vi "Channel Calibration.vi"(8 "error in (no error)":errorcluster, 9 "Gain":dbl, 10 "Channel Name":string, 11 "index":i32) -> (0 "error out":errorcluster, 1 "Offset":dbl, 2 "Gain":dbl, 3 "Status Output":T1)   [LabVIEW 2011]
uses:
  Calibration SubVIs/Controls/typedef_enum_Calibration Type.ctl
  Controls/typedef_enum_Calibration SM States.ctl
  Calibration SubVIs/Controls/typedef_enum_GFV Calibration GUI_actions.ctl
  Controls/typedef_cluster_Calibration Status.ctl
  Measurments Handling/Action Analog Handler.ctl
panel:
  out "Waveform Chart":dbl(graph)
  in  "Cancel":bool
  in  "OK":bool
  out "Instructions":string
  in  "Back":bool
  in  "Next":bool
  in  "Calibration Type":T2
  out "X2":dbl
  in  "Y2":dbl
  out "X1":dbl
  in  "Y1":dbl
  # "Channel Calibration"
  # "1st point"
  # "2nd point"
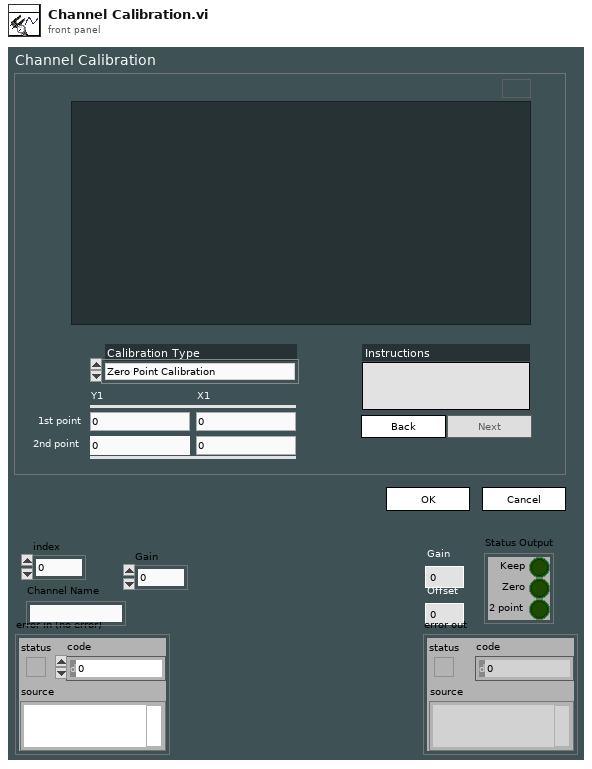
[diagram p1: front panel]
types:
  T1 = cluster{"Keep":bool, "Zero":bool, "2 point":bool}
  T2 = typedef "typedef_enum_Calibration Type.ctl" = enum16{"Zero Point Calibration", "Two Point Calibration"}
  T3 = typedef "typedef_cluster_Calibration Status.ctl" = cluster{"Keep":bool, "Zero":bool, "2 point":bool}
  T4 = typedef "typedef_enum_Calibration SM States.ctl" = enum16{"Idle", "Init", "2 pnt Enter 1st", "2 pnt Measure 1st", "2 pnt Enter 2nd", "2 pnt Measure 2nd", "2 pnt Calculate", "Zero Measure", "Zero Calculate", "Increment", "Decrement"}
  T5 = typedef "typedef_enum_GFV Calibration GUI_actions.ctl" = enum16{"Init", "Update GUI", "Clear GUI"}
  T6 = enum8{"Enabled", "Disabled", "Disabled and Grayed Out"}
  T7 = typedef "Action Analog Handler.ctl" = enum16{"GET value", "GET Single Frequenzy", "GET All Values", "GET Waveform", "Get Numb Var", "SET Value", "START Buffer", "REG Variable", "BUF size(total antal sekund)", "PULS", "Get a Value at time", "Set initial waveform"}
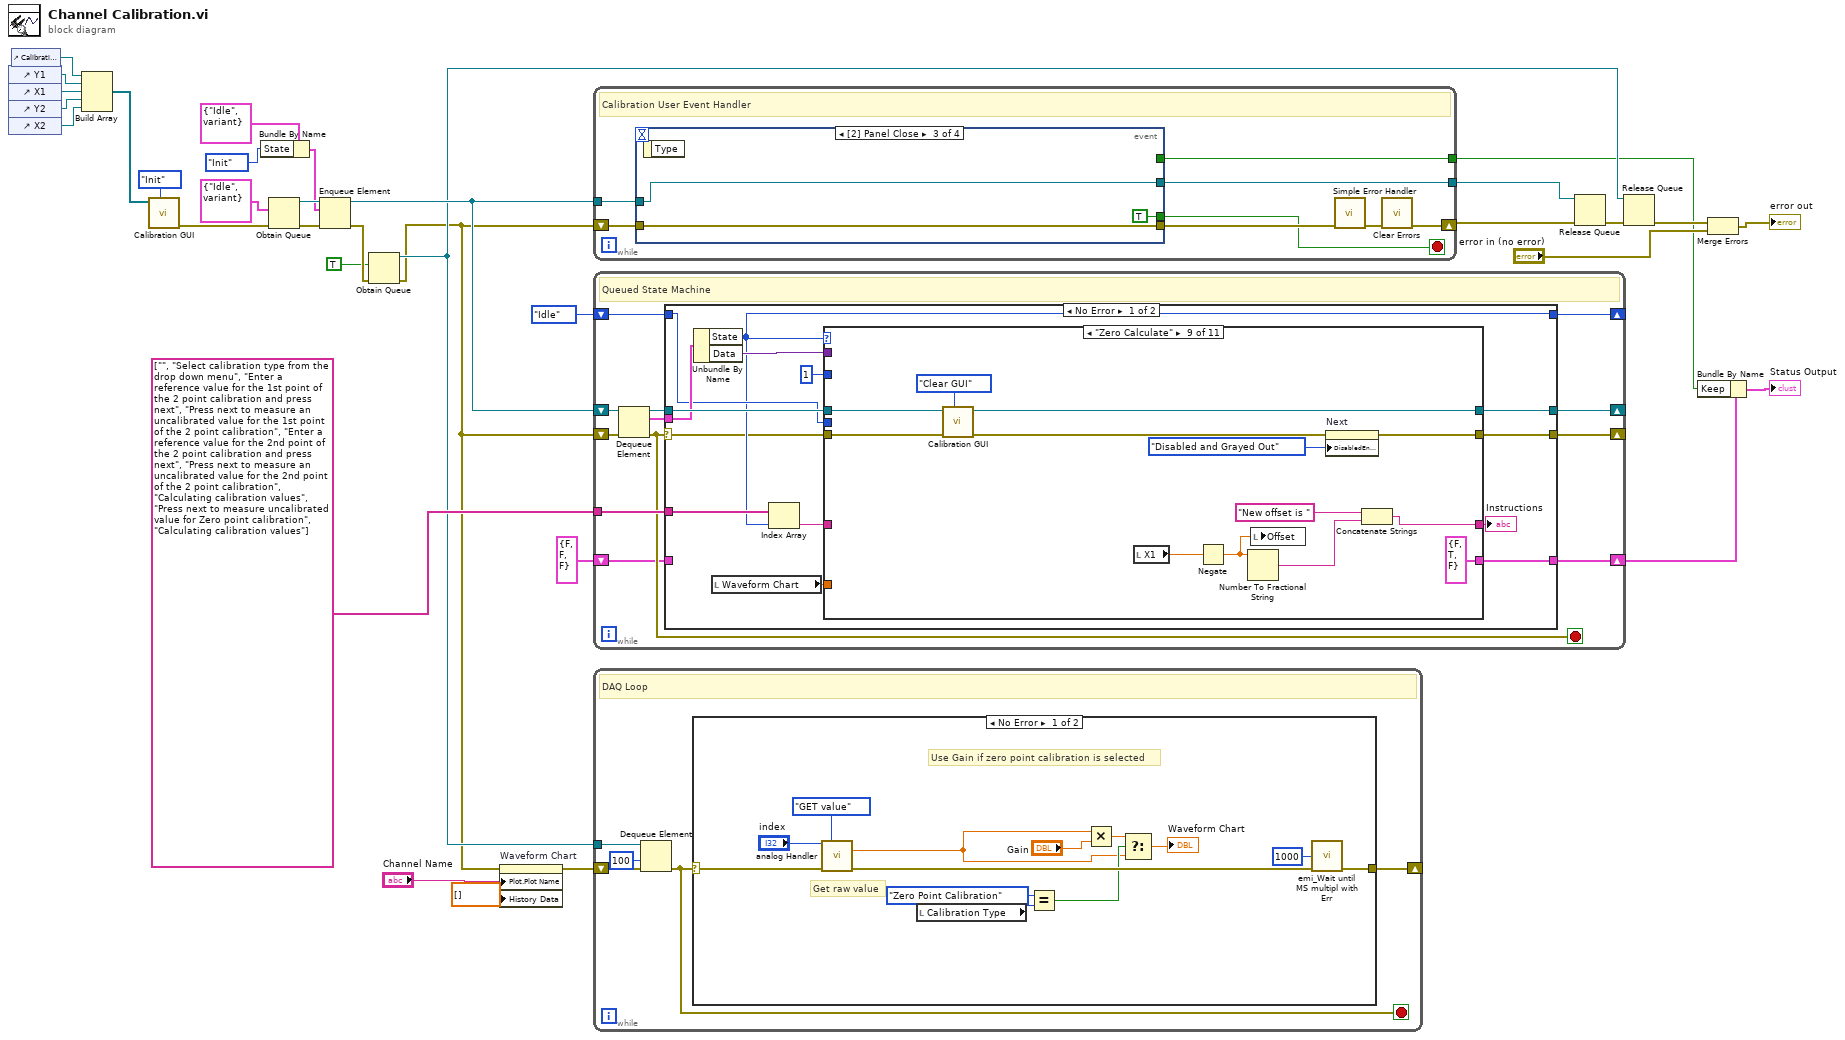
[diagram p0: block diagram]
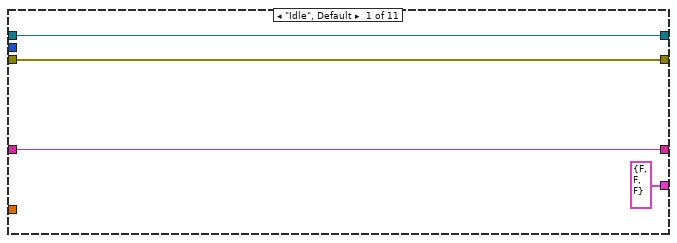
[diagram p3: hidden frame]
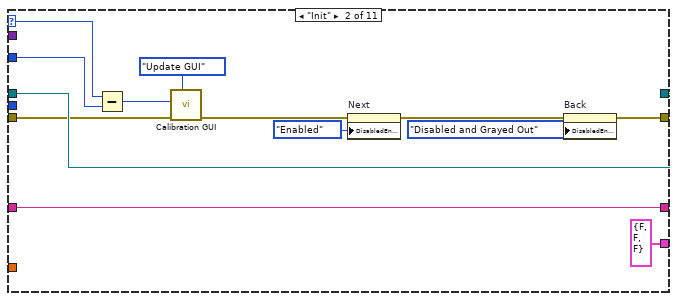
[diagram p4: hidden frame]
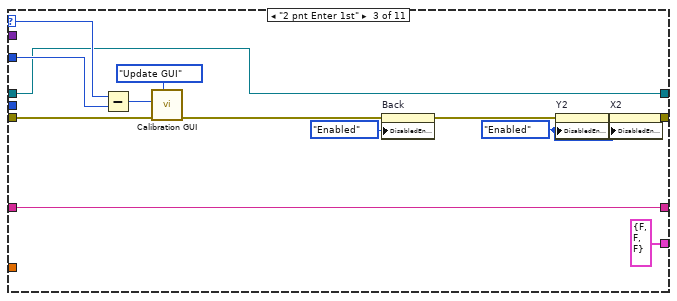
[diagram p5: hidden frame]
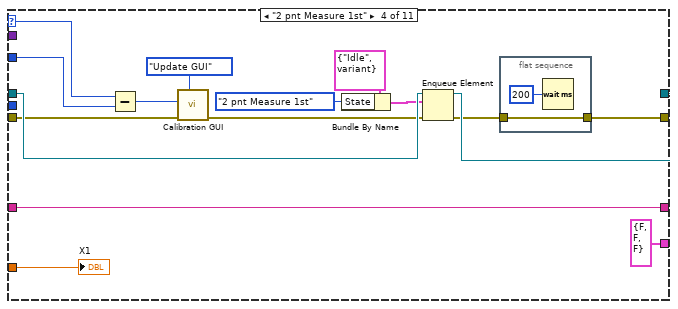
[diagram p6: hidden frame]
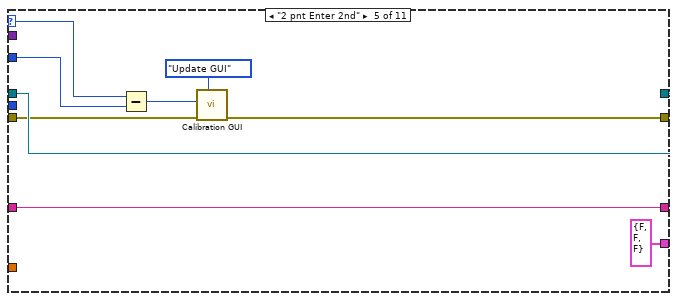
[diagram p7: hidden frame]
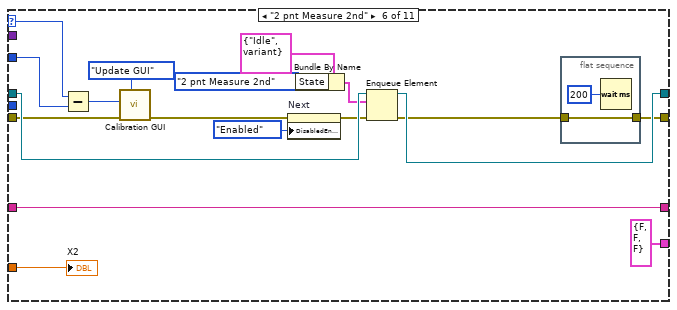
[diagram p8: hidden frame]
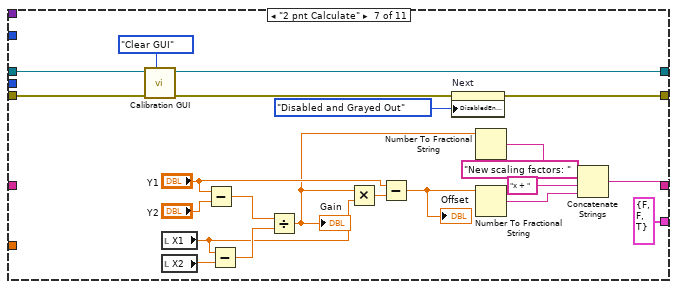
[diagram p9: hidden frame]
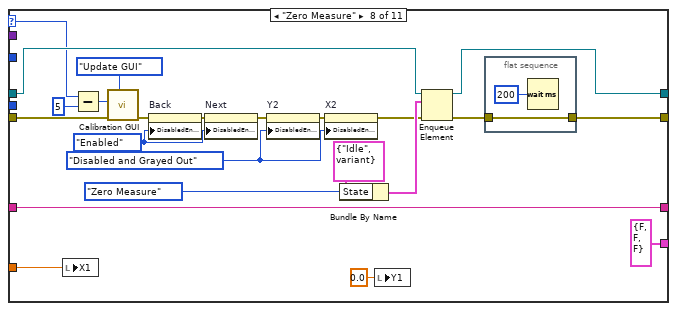
[diagram p10: hidden frame]
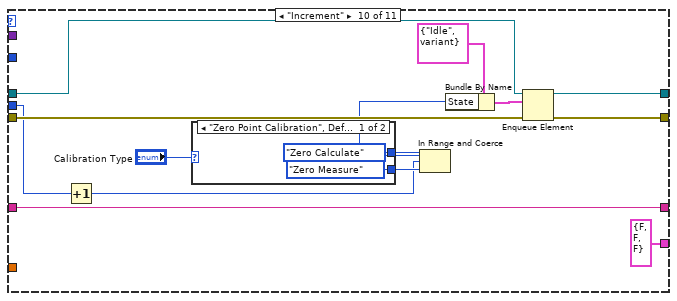
[diagram p11: hidden frame]
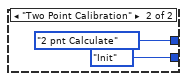
[diagram p12: hidden frame]
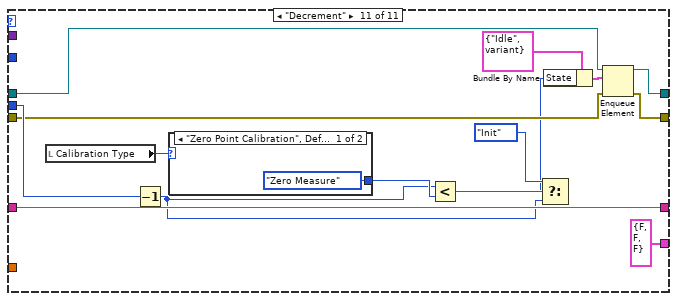
[diagram p13: hidden frame]
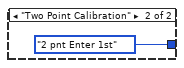
[diagram p14: hidden frame]
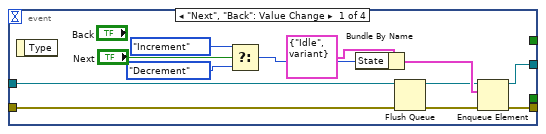
[diagram p16: hidden frame]
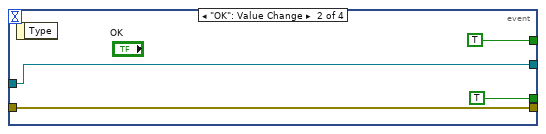
[diagram p17: hidden frame]
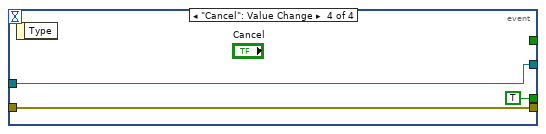
[diagram p18: hidden frame]
diagram:
  n1 = control-ref of="Y1"() -> (w29:refnum<vi>)
  n2 = control-ref of="X1"() -> (w28:refnum<vi>)
  n3 = control-ref of="Y2"() -> (w27:refnum<vi>)
  n4 = control-ref of="X2"() -> (w26:refnum<vi>)
  n5 = control-ref of="Calibration Type"() -> (w18:refnum<vi>)
  n6 = Build Array(w18, w29, w28, w27, w26) -> (w25:refnum<vi>[])
  n7 = call "Calibration GUI.vi"("Actions"=typedef_enum_GFV_Calibration_GUI_actions."Init", "Ctrl Ref"=w25) -> ("error out"=w30:errorcluster)  [unwired: 9 in]
  n8 = Bundle By Name(cluster=cluster{"State":T4, "Data":variant} {"State"=enum."Idle", "Data"=variant} ("element"), "State"=typedef_enum_Calibration_SM_States."Init") -> (w20:cluster{"State":T4, "Data":variant})
  n9 = Obtain Queue(element data type=cluster{"State":T4, "Data":variant} {"State"=enum."Idle", "Data"=variant} ("Cluster"), error in (no error)=w30) -> (queue out=w24:refnum<queue>, error out=w22:errorcluster)  [unwired: 3 in, 1 out]
  n10 = Enqueue Element(queue=w24, element=w20, error in (no error)=w22) -> (queue out=w23:refnum<queue>, error out=w13:errorcluster)  [unwired: 1 in, 1 out]
  n11 = Obtain Queue(element data type=TRUE, error in (no error)=w13) -> (queue out=w9:refnum<queue>, error out=w3:errorcluster)  [unwired: 3 in, 1 out]
  n12 = property on="Waveform Chart" class="WFChart (strict)"(error in=w3, "Plot.Plot Name"="Channel Name", "History Data"=dbl[] []) -> (error out=w2:errorcluster)  [unwired: 1 in, 1 out]
  n13 = while {
    tunnel: w23 -> [w42]
    shift-right: [w38] -> w16
    shift-left: w3 -> [w41]
    tunnel: [w37] -> w17
    tunnel: [w35] -> w7
    stop <- w36 stop-if-true
    # "Calibration User Event Handler"
    n14 = event shown="[2] Panel Close" {
      selector: _ -> [_ _ _ _]
      dyn-events: _ -> [_ _ _ _]
      timeout: _ -> [_ _ _ _]
      tunnel: w42 -> [w52 w58 w61 w64]
      tunnel: w41 -> [w46 w57 w60 w63]
      tunnel: [w44 w57 w60 w63] -> w40
      tunnel: [w43 w58 w61 w64] -> w37
      tunnel: [_ TRUE TRUE TRUE] -> w36
      tunnel: [_ TRUE _ _] -> w35
      event "Next", "Back": Value Change {
        n15 = event-data() -> ()  [unwired: 1 in, 1 out]
        n16 = Select(t=typedef_enum_Calibration_SM_States."Increment" ("State"), s="Next", f=typedef_enum_Calibration_SM_States."Decrement") -> (s? t:f=w48:T4)
        n17 = Bundle By Name(cluster=cluster{"State":T4, "Data":variant} {"State"=enum."Idle", "Data"=variant} ("Cluster"), "State"=w48) -> (w53:cluster{"State":T4, "Data":variant})
        n18 = Flush Queue(queue=w52, error in (no error)=w46) -> (queue out=w51:refnum<queue>, error out=w45:errorcluster)  [unwired: 1 out]
        n19 = Enqueue Element(queue=w51, element=w53, error in (no error)=w45) -> (queue out=w43:refnum<queue>, error out=w44:errorcluster)  [unwired: 1 in, 1 out]
      }
      event "OK": Value Change {
        n20 = event-data() -> ()  [unwired: 1 in, 1 out]
      }
      event Panel Close {
        n21 = event-data() -> ()  [unwired: 1 in, 1 out]
      }
      event "Cancel": Value Change {
        n22 = event-data() -> ()  [unwired: 1 in, 1 out]
      }
    }
    n23 = call <vilib>:"Simple Error Handler.vi"("error in (no error)"=w40) -> ("error out"=w39:errorcluster)  [unwired: 4 in, 4 out]
    n24 = call <vilib>:"Clear Errors.vi"("error in (no error)"=w39) -> ("error out"=w38:errorcluster)  [unwired: 6 in]
  }
  n25 = while {
    shift-right: [w72] -> _
    shift-left: w23 -> [w76]
    shift-right: [w71] -> _
    shift-left: w3 -> [w75]
    shift-right: [w68] -> _
    shift-left: typedef_enum_Calibration_SM_States."Idle" ("State") -> [w70]
    tunnel: string[] ["", "Select calibration type from the drop down menu", "Enter a reference value for the 1st point of the 2 point calibration and press next", "Press next to measure an uncalibrated value for the 1st point of the 2 point calibration", "Enter a reference value for the 2nd point of the 2 point calibration and press next", "Press next to measure an uncalibrated value for the 2nd point of the 2 point calibration", "Calculating calibration values", "Press next to measure uncalibrated value for Zero point calibration", "Calculating calibration values"] -> [w69]
    shift-right: [w65] -> w5
    shift-left: T3 {"Keep"=FALSE, "Zero"=FALSE, "2 point"=FALSE} ("Status Output") -> [w66]
    stop <- w67 stop-if-true
    # "Queued State Machine"
    n26 = Dequeue Element(queue=w76, error in (no error)=w75) -> (queue out=w74:refnum<queue>, element=w73:cluster{"State":T4, "Data":variant}, error out=w67:errorcluster)  [unwired: 1 in, 1 out]
    n27 = case shown="No Error" w67 {
      selector: w67 -> [w78 w263]
      tunnel: w74 -> [w90 w264]
      tunnel: w73 -> [w89 _]
      tunnel: [w87 w264] -> w72
      tunnel: [w86 w263] -> w71
      tunnel: w70 -> [w85 w265]
      tunnel: w69 -> [w84 _]
      tunnel: [w81 w265] -> w68
      tunnel: w66 -> [_ w262]
      tunnel: [w77 w262] -> w65
      frame No Error {
        n28 = Unbundle By Name(w89) -> ("State"=w81:T4, "Data"=w88:variant)
        n29 = local read "Waveform Chart"() -> (w83:dbl)
        n30 = Index Array(array=w84, index=w81) -> (element=w80:string)
        n31 = case shown="\"Zero Calculate\"" w81 {
          selector: w81 -> [_ w104 w121 w133 w147 w164 _ w201 _ _ _]
          tunnel: w90 -> [w94 w107 w111 w137 w148 w165 w182 w203 w224 w240 w259]
          tunnel: w78 -> [w93 w96 w113 w126 w142 w153 w172 w206 w222 w236 w254]
          tunnel: w88 -> [_ _ _ _ _ _ _ _ _ _ _]
          tunnel: [w94 w107 w111 w135 w148 w166 w182 w204 w224 w239 w258] -> w87
          tunnel: [w93 w97 w112 w124 w141 w151 w174 w205 w225 w235 w253] -> w86
          tunnel: w83 -> [_ _ _ w123 _ w150 _ w191 _ _ _]
          tunnel: w85 -> [_ _ _ _ _ _ _ _ _ w231 w257]
          tunnel: 1 -> [_ w103 w118 w128 w144 w158 _ _ _ _ _]
          tunnel: w80 -> [w92 w102 w117 w127 w143 w157 _ w212 _ w233 w252]
          tunnel: [w92 w102 w117 w127 w143 w157 w176 w212 w217 w233 w252] -> w79
          tunnel: [T3 {"Keep"=FALSE, "Zero"=FALSE, "2 point"=FALSE} ("Status Output") T3 {"Keep"=FALSE, "Zero"=FALSE, "2 point"=FALSE} ("Status Output") T3 {"Keep"=FALSE, "Zero"=FALSE, "2 point"=FALSE} ("Status Output") T3 {"Keep"=FALSE, "Zero"=FALSE, "2 point"=FALSE} ("Status Output") T3 {"Keep"=FALSE, "Zero"=FALSE, "2 point"=FALSE} ("Status Output") T3 {"Keep"=FALSE, "Zero"=FALSE, "2 point"=FALSE} ("Status Output") T3 {"Keep"=FALSE, "Zero"=FALSE, "2 point"=TRUE} ("Status Output") T3 {"Keep"=FALSE, "Zero"=FALSE, "2 point"=FALSE} ("Status Output") T3 {"Keep"=FALSE, "Zero"=TRUE, "2 point"=FALSE} ("Status Output") T3 {"Keep"=FALSE, "Zero"=FALSE, "2 point"=FALSE} ("Status Output") T3 {"Keep"=FALSE, "Zero"=FALSE, "2 point"=FALSE} ("Status Output")] -> w77
          frame "Idle", Default {
          }
          frame "Init" {
            n32 = Subtract(x=w104, y=w103) -> (x-y=w105:i32)
            n33 = call "Calibration GUI.vi"("Actions"=typedef_enum_GFV_Calibration_GUI_actions."Update GUI", "error in (no error)"=w96, "index"=w105) -> ("error out"=w99:errorcluster)  [unwired: 8 in]
            n34 = property on="Next" class="Bool"(error in=w99, "DisabledEnum"=T6."Enabled" ("Disabled")) -> (error out=w98:errorcluster)  [unwired: 1 in, 1 out]
            n35 = property on="Back" class="Bool"(error in=w98, "DisabledEnum"=T6."Disabled and Grayed Out" ("Disabled")) -> (error out=w97:errorcluster)  [unwired: 1 in, 1 out]
          }
          frame "2 pnt Enter 1st" {
            w109 = T6."Enabled" ("Disabled")
            n36 = Subtract(x=w121, y=w118) -> (x-y=w119:i32)
            n37 = call "Calibration GUI.vi"("Actions"=typedef_enum_GFV_Calibration_GUI_actions."Update GUI", "error in (no error)"=w113, "index"=w119) -> ("error out"=w114:errorcluster)  [unwired: 8 in]
            n38 = property on="Back" class="Bool"(error in=w114, "DisabledEnum"=T6."Enabled" ("Disabled")) -> (error out=w115:errorcluster)  [unwired: 1 in, 1 out]
            n39 = property on="Y2" class="DigNum (strict)"(error in=w115, "DisabledEnum"=w109) -> (error out=w110:errorcluster)  [unwired: 1 in, 1 out]
            n40 = property on="X2" class="DigNum (strict)"(error in=w110, "DisabledEnum"=w109) -> (error out=w112:errorcluster)  [unwired: 1 in, 1 out]
          }
          frame "2 pnt Measure 1st" {
            n41 = Subtract(x=w133, y=w128) -> (x-y=w130:i32)
            n42 = call "Calibration GUI.vi"("Actions"=typedef_enum_GFV_Calibration_GUI_actions."Update GUI", "error in (no error)"=w126, "index"=w130) -> ("error out"=w125:errorcluster)  [unwired: 8 in]
            n43 = Bundle By Name(cluster=cluster{"State":T4, "Data":variant} {"State"=enum."Idle", "Data"=variant} ("element"), "State"=typedef_enum_Calibration_SM_States."2 pnt Measure 1st") -> (w131:cluster{"State":T4, "Data":variant})
            n44 = Enqueue Element(queue=w137, element=w131, error in (no error)=w125) -> (queue out=w135:refnum<queue>, error out=w134:errorcluster)  [unwired: 1 in, 1 out]
            n45 = flat-sequence {
              tunnel: w134 -> [w138]
              tunnel: [w138] -> w124
              frame #0 {
                n46 = Wait (ms)(milliseconds to wait=u32 200) -> ()  [unwired: 1 out]
              }
            }
            "X1" <- w123
          }
          frame "2 pnt Enter 2nd" {
            n47 = Subtract(x=w147, y=w144) -> (x-y=w146:i32)
            n48 = call "Calibration GUI.vi"("Actions"=typedef_enum_GFV_Calibration_GUI_actions."Update GUI", "error in (no error)"=w142, "index"=w146) -> ("error out"=w141:errorcluster)  [unwired: 8 in]
          }
          frame "2 pnt Measure 2nd" {
            n49 = Subtract(x=w164, y=w158) -> (x-y=w160:i32)
            n50 = call "Calibration GUI.vi"("Actions"=typedef_enum_GFV_Calibration_GUI_actions."Update GUI", "error in (no error)"=w153, "index"=w160) -> ("error out"=w155:errorcluster)  [unwired: 8 in]
            n51 = property on="Next" class="Bool"(error in=w155, "DisabledEnum"=T6."Enabled" ("Disabled")) -> (error out=w154:errorcluster)  [unwired: 1 in, 1 out]
            n52 = Bundle By Name(cluster=cluster{"State":T4, "Data":variant} {"State"=enum."Idle", "Data"=variant} ("element"), "State"=typedef_enum_Calibration_SM_States."2 pnt Measure 2nd") -> (w162:cluster{"State":T4, "Data":variant})
            n53 = Enqueue Element(queue=w165, element=w162, error in (no error)=w154) -> (queue out=w166:refnum<queue>, error out=w152:errorcluster)  [unwired: 1 in, 1 out]
            n54 = flat-sequence {
              tunnel: w152 -> [w167]
              tunnel: [w167] -> w151
              frame #0 {
                n55 = Wait (ms)(milliseconds to wait=u32 200) -> ()  [unwired: 1 out]
              }
            }
            "X2" <- w150
          }
          frame "2 pnt Calculate" {
            n56 = call "Calibration GUI.vi"("Actions"=typedef_enum_GFV_Calibration_GUI_actions."Clear GUI", "error in (no error)"=w172) -> ("error out"=w171:errorcluster)  [unwired: 9 in]
            n57 = local read "X1"() -> (w186:dbl)
            n58 = local read "X2"() -> (w189:dbl)
            n59 = Subtract(x="Y1", y="Y2") -> (x-y=w188:dbl)
            n60 = Subtract(x=w186, y=w189) -> (x-y=w187:dbl)
            n61 = Divide(x=w188, y=w187) -> (x/y=w181:dbl)
            "Gain" <- w181
            n62 = Multiply(x=w181, y=w186) -> (x*y=w185:dbl)
            n63 = Subtract(x="Y1", y=w185) -> (x-y=w180:dbl)
            "Offset" <- w180
            n64 = property on="Next" class="Bool"(error in=w171, "DisabledEnum"=T6."Disabled and Grayed Out" ("Disabled")) -> (error out=w174:errorcluster)  [unwired: 1 in, 1 out]
            n65 = Number To Fractional String(number=w181) -> (F-format string=w179:string)  [unwired: 3 in]
            n66 = Number To Fractional String(number=w180) -> (F-format string=w177:string)  [unwired: 3 in]
            n67 = Concatenate Strings("New scaling factors: " ("string"), w179, "x + " ("string"), w177) -> (w176:string)
          }
          frame "Zero Measure" {
            w192 = T6."Enabled" ("Disabled")
            w198 = T6."Disabled and Grayed Out" ("Disabled")
            n68 = local write "X1"(w191) -> ()
            n69 = Subtract(x=w201, y=5) -> (x-y=w208:i32)
            n70 = call "Calibration GUI.vi"("Actions"=typedef_enum_GFV_Calibration_GUI_actions."Update GUI", "error in (no error)"=w206, "index"=w208) -> ("error out"=w194:errorcluster)  [unwired: 8 in]
            n71 = property on="Back" class="Bool"(error in=w194, "DisabledEnum"=w192) -> (error out=w193:errorcluster)  [unwired: 1 in, 1 out]
            n72 = property on="Next" class="Bool"(error in=w193, "DisabledEnum"=w192) -> (error out=w196:errorcluster)  [unwired: 1 in, 1 out]
            n73 = property on="Y2" class="DigNum (strict)"(error in=w196, "DisabledEnum"=w198) -> (error out=w199:errorcluster)  [unwired: 1 in, 1 out]
            n74 = property on="X2" class="DigNum (strict)"(error in=w199, "DisabledEnum"=w198) -> (error out=w195:errorcluster)  [unwired: 1 in, 1 out]
            n75 = Bundle By Name(cluster=cluster{"State":T4, "Data":variant} {"State"=enum."Idle", "Data"=variant} ("element"), "State"=typedef_enum_Calibration_SM_States."Zero Measure") -> (w209:cluster{"State":T4, "Data":variant})
            n76 = local write "Y1"(0.0 ("Y1")) -> ()
            n77 = Enqueue Element(queue=w203, element=w209, error in (no error)=w195) -> (queue out=w204:refnum<queue>, error out=w210:errorcluster)  [unwired: 1 in, 1 out]
            n78 = flat-sequence {
              tunnel: w210 -> [w213]
              tunnel: [w213] -> w205
              frame #0 {
                n79 = Wait (ms)(milliseconds to wait=u32 200) -> ()  [unwired: 1 out]
              }
            }
          }
          frame "Zero Calculate" {
            n80 = call "Calibration GUI.vi"("Actions"=typedef_enum_GFV_Calibration_GUI_actions."Clear GUI", "error in (no error)"=w222) -> ("error out"=w221:errorcluster)  [unwired: 9 in]
            n81 = local read "X1"() -> (w219:dbl)
            n82 = Negate(x=w219) -> (-x=w216:dbl)
            n83 = Number To Fractional String(number=w216) -> (F-format string=w220:string)  [unwired: 3 in]
            n84 = local write "Offset"(w216) -> ()
            n85 = property on="Next" class="Bool"(error in=w221, "DisabledEnum"=T6."Disabled and Grayed Out" ("Disabled")) -> (error out=w225:errorcluster)  [unwired: 1 in, 1 out]
            n86 = Concatenate Strings("New offset is " ("string"), w220) -> (w217:string)
          }
          frame "Increment" {
            n87 = Increment(x=w231) -> (x+1=w228:T4)
            n88 = case shown="\"Zero Point Calibration\", Default" "Calibration Type" {
              tunnel: [typedef_enum_Calibration_SM_States."Zero Calculate" ("upper limit") typedef_enum_Calibration_SM_States."2 pnt Calculate" ("upper limit")] -> w230
              tunnel: [typedef_enum_Calibration_SM_States."Zero Measure" ("lower limit") typedef_enum_Calibration_SM_States."Init" ("lower limit")] -> w229
              frame "Zero Point Calibration", Default {
              }
              frame "Two Point Calibration" {
              }
            }
            n89 = In Range and Coerce(upper limit=w230, x=w228, lower limit=w229) -> (coerced(x)=w234:T4)  [unwired: 1 out]
            n90 = Bundle By Name(cluster=cluster{"State":T4, "Data":variant} {"State"=enum."Idle", "Data"=variant} ("element"), "State"=w234) -> (w237:cluster{"State":T4, "Data":variant})
            n91 = Enqueue Element(queue=w240, element=w237, error in (no error)=w236) -> (queue out=w239:refnum<queue>, error out=w235:errorcluster)  [unwired: 1 in, 1 out]
          }
          frame "Decrement" {
            n92 = local read "Calibration Type"() -> (w251:T2)
            n93 = Decrement(x=w257) -> (x-1=w246:T4)
            n94 = case shown="\"Zero Point Calibration\", Default" w251 {
              tunnel: [typedef_enum_Calibration_SM_States."Zero Measure" ("lower limit") typedef_enum_Calibration_SM_States."2 pnt Enter 1st" ("lower limit")] -> w247
              frame "Zero Point Calibration", Default {
              }
              frame "Two Point Calibration" {
              }
            }
            n95 = Less?(x=w246, y=w247) -> (x < y?=w250:bool)
            n96 = Select(t=typedef_enum_Calibration_SM_States."Init" ("lower limit"), s=w250, f=w246) -> (s? t:f=w248:T4)
            n97 = Bundle By Name(cluster=cluster{"State":T4, "Data":variant} {"State"=enum."Idle", "Data"=variant} ("element"), "State"=w248) -> (w255:cluster{"State":T4, "Data":variant})
            n98 = Enqueue Element(queue=w259, element=w255, error in (no error)=w254) -> (queue out=w258:refnum<queue>, error out=w253:errorcluster)  [unwired: 1 in, 1 out]
          }
        }
        "Instructions" <- w79
      }
      frame Error {
      }
    }
  }
  n99 = while {
    shift-right: [w270] -> _
    shift-left: w2 -> [w269]
    tunnel: w9 -> [w268]
    stop <- w266 stop-if-true
    # "DAQ Loop"
    n100 = Dequeue Element(queue=w268, timeout in ms (-1)=100, error in (no error)=w269) -> (error out=w266:errorcluster)  [unwired: 3 out]
    n101 = case shown="No Error" w266 {
      selector: w266 -> [w280 w284]
      tunnel: [w282 w284] -> w270
      frame No Error {
        # "Use Gain if zero point calibration is selected"
        # "Get raw value"
        n102 = call "analog Handler.vi"("Variable Index"="index", "Action"=Action_Analog_Handler."GET value" ("Action(GET)"), "error in (no error)"=w280) -> ("Value out"=w272:dbl, "error out"=w279:errorcluster)  [unwired: 7 in, 4 out]
        n103 = local read "Calibration Type"() -> (w276:T2)
        n104 = Equal?(x=typedef_enum_Calibration_Type."Zero Point Calibration", y=w276) -> (x = y?=w274:bool)
        n105 = Multiply(x=w272, y="Gain") -> (x*y=w273:dbl)
        n106 = Select(t=w273, s=w274, f=w272) -> (s? t:f=→"Waveform Chart":dbl)
        n107 = call "emi_Wait until MS multipl with Err.vi"("millisecond multiple(0)"=u32 1000, "error in (no error)"=w279) -> ("error out"=w282:errorcluster)  [unwired: 13 in]
      }
      frame Error {
      }
    }
  }
  n108 = Release Queue(queue=w17, error in (no error)=w16) -> (error out=w11:errorcluster)  [unwired: 1 in, 2 out]
  n109 = Release Queue(queue=w9, error in (no error)=w11) -> (error out=w10:errorcluster)  [unwired: 1 in, 2 out]
  n110 = Bundle By Name(cluster=w5, "Keep"=w7) -> (→"Status Output":T3)
  n111 = Merge Errors(w10, "error in (no error)") -> (→"error out":errorcluster)
